vi "Lidar Code XY - Minimal.vi"() -> ()   [LabVIEW 2016]
uses:
  <instrlib>/Hokuyo URG Series/Public/Initialize-cRIO-USB.vi
  <instrlib>/Hokuyo URG Series/Hokuyo URG Series.lvlib
panel:
  out "XY Graph 1.5m max":cluster{"Y":dbl[], "Y":dbl[]}[](graph)
  out "XY Graph 6m max":cluster{"Y":dbl[], "Y":dbl[]}[](graph)
  in  "Protocol":u32(ring)=2 items=["Convert to Latest", "SCIP 1.1", "SCIP 2.0"]
  in  "ID Query?":bool=TRUE
  in  "Checksum":bool
  in  "Stop":bool
  in  "End Point":dbl=120.0
  in  "Start Point":dbl=-120.0
  in  "Cluster Count":dbl=1.0
  in  "Encoding Width":u16(ring)=3 items=["2 Byte"=2, "3 Byte"=3]
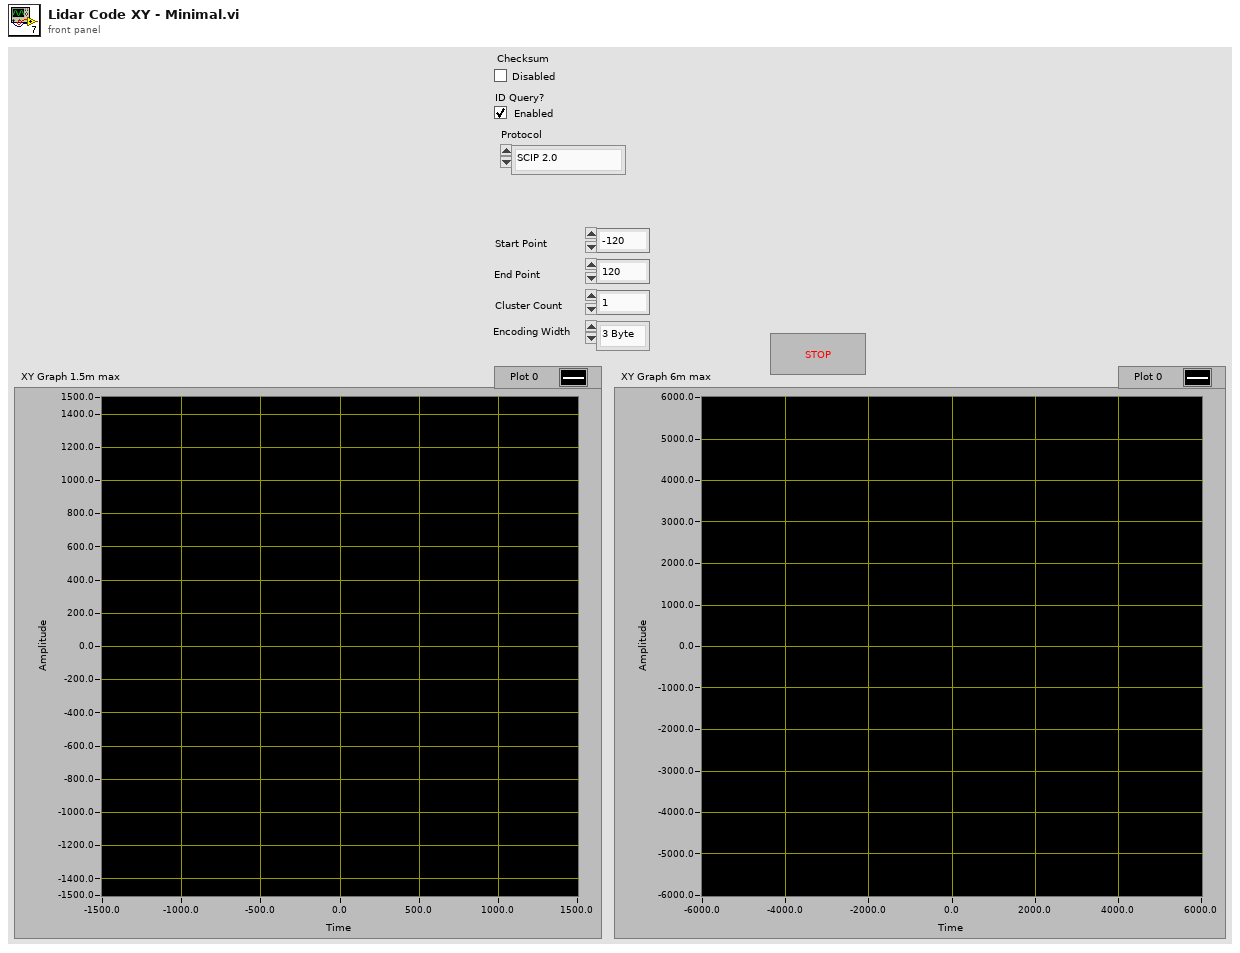
[diagram p1: front panel]
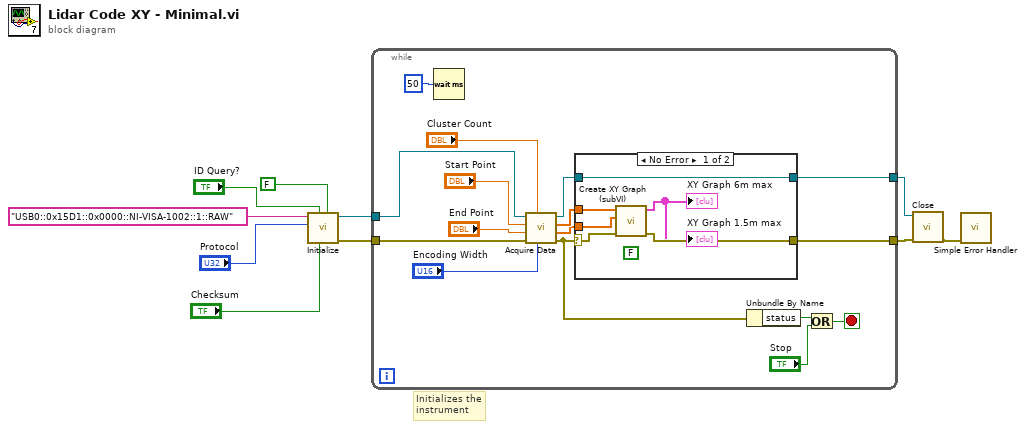
[diagram p0: block diagram]
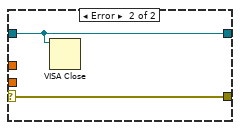
[diagram p2: hidden frame]
diagram:
  # "Initializes the instrument"
  n1 = call-poly <instrlib>:"Initialize.vi"("Reset? (F: No)"=FALSE ("Reset Instrument (Disabled)"), "Checksum (Disabled)"="Checksum", "ID Query? (Enabled)"="ID Query?", "Protocol (2: SCIP 2.0)"="Protocol", "VISA resource name"="USB0::0x15D1::0x0000::NI-VISA-1002::1::RAW") -> ("error out"=w3:errorcluster, "VISA resource name out"=w4:refnum<visa-resource-name>)  [unwired: 5 in]
  n2 = while {
    tunnel: w4 -> [w16]
    tunnel: [w12] -> w10
    tunnel: w3 -> [w15]
    tunnel: [w11] -> w1
    stop <- w24 stop-if-true
    n3 = Wait (ms)(milliseconds to wait=u32 50) -> ()  [unwired: 1 out]
    n4 = call <instrlib>:"Acquire Data.vi"("Data Encoding Width (3 Byte)"="Encoding Width", "Cluster Count (1)"="Cluster Count", "error in (no error)"=w15, "End Point (120°)"="End Point", "Start Point (-120°)"="Start Point", "VISA resource name"=w16) -> ("error out"=w20:errorcluster, "Direction"=w21:dbl[], "Magnitude"=w22:dbl[], "VISA resource name out"=w23:refnum<visa-resource-name>)  [unwired: 2 in]
    n5 = case shown="No Error" w20 {
      selector: w20 -> [w29 w34]
      tunnel: [w28 w34] -> w12
      tunnel: w23 -> [w32 w33]
      tunnel: [w32 w33] -> w11
      tunnel: w22 -> [w30 _]
      tunnel: w21 -> [w31 _]
      frame No Error {
        (unwired) FALSE
        n6 = call "Create XY Graph (subVI).vi"("error in"=w29, "Direction"=w31, "Magnitude"=w30) -> ("error out"=w28:errorcluster, "XY Graph"=→"XY Graph 1.5m max" →"XY Graph 6m max":cluster{"Y":dbl[], "Y":dbl[]}[])  [unwired: 6 in, 1 out]
      }
      frame Error {
        n7 = VISA Close(VISA resource name=w33) -> ()  [unwired: 1 in, 1 out]
      }
    }
    n8 = Unbundle By Name(w20) -> ("status"=w26:bool)
    n9 = Or(x=w26, y="Stop") -> (x .or. y?=w24:bool)
  }
  n10 = call <instrlib>:"Close.vi"("error in (no error)"=w10, "VISA resource name"=w1) -> ("error out"=w8:errorcluster)  [unwired: 9 in]
  n11 = call <vilib>:"Simple Error Handler.vi"("error in (no error)"=w8) -> ()  [unwired: 4 in, 5 out]
